vi "Set Channel Value Table.vi"(8 "error in (no error)":errorcluster, 9 "Values":dbl[](array[numeric]), 10 "States":string[](array[string]), 11 "Channel Ref in":T1 format="%.0x") -> (0 "error out":errorcluster, 3 "Channel Ref out":T1=18446744073709551615 format="%.0x")   [LabVIEW 2017, in "Switch Scripting.lvlib"]
uses:
  Switch Scripting.lvlib
  <vilib>/NI Veristand/Custom Device API/Custom Device Item Ref.ctl
  NationalInstruments.VeriStand.SystemDefinitionAPI
  NationalInstruments.VeriStand.SystemStorage
  <vilib>/NI VeriStand/Custom Device API/Custom Device API.lvlib
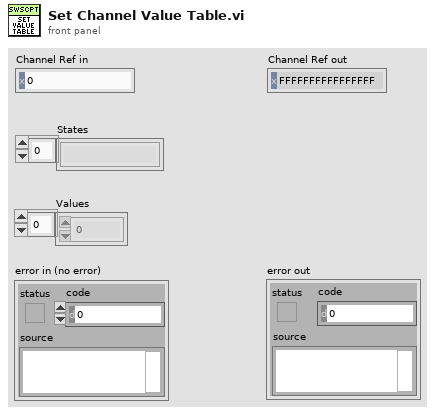
[diagram p1: front panel]
types:
  T1 = typedef "Custom Device API.lvlib/Custom Device Item Ref.ctl" = u64
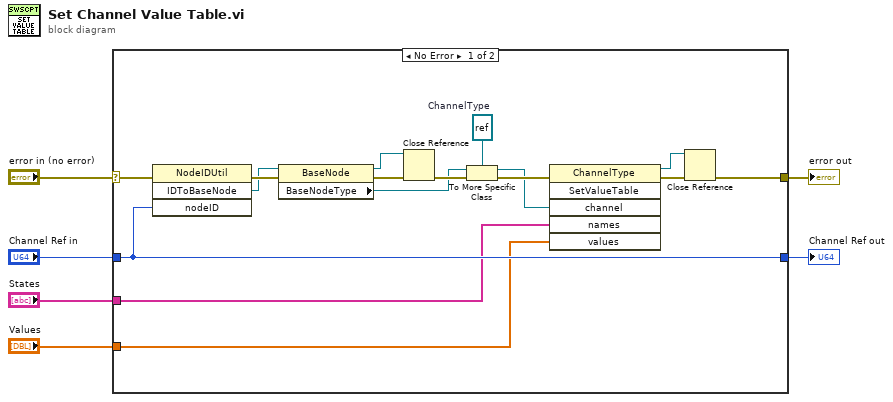
[diagram p0: block diagram]
diagram:
  n1 = case shown="No Error" "error in (no error)" {
    selector: "error in (no error)" -> [w19 w24]
    tunnel: [w18 w24] -> w5
    tunnel: "Channel Ref in" -> [w17 w23]
    tunnel: [w17 w23] -> w3
    tunnel: "States" -> [w9 _]
    tunnel: "Values" -> [w8 _]
    frame No Error {
      w15 = refnum<k24> refnum  # ChannelType
      n2 = invoke class="NodeIDUtil" method="IDToBaseNode"(error in=w19, "nodeID"=w17) -> (error out=w22:errorcluster, "IDToBaseNode"=w20:refnum<k24>)  [unwired: 2 in, 2 out]
      n3 = property class="BaseNode"(reference=w20, error in=w22) -> (reference out=w7:refnum<k24>, error out=w21:errorcluster, "BaseNodeType"=w12:refnum<k24>)
      n4 = Close Reference(reference=w7, error in (no error)=w21) -> (error out=w13:errorcluster)
      n5 = To More Specific Class(target class=w15, reference=w12, error in=w13) -> (specific class reference=w14:refnum<k24>, error out=w16:errorcluster)
      n6 = invoke class="ChannelType" method="SetValueTable"(error in=w16, "channel"=w14, "names"=w9, "values"=w8) -> (reference out=w10:refnum<k24>, error out=w11:errorcluster)  [unwired: 2 in, 4 out]
      n7 = Close Reference(reference=w10, error in (no error)=w11) -> (error out=w18:errorcluster)
    }
    frame Error {
    }
  }
  "Channel Ref out" <- w3
  "error out" <- w5
